vi "scope_stats.vi"(0 "Data Save":path[](array[path]), 1 "Seq":string, 4 "Save Array":bool[](array[boolean]), 5 "ext":string=".ch_a#", 6 "Repeat":u32=5, 7 "Save All":bool, 8 "Waveform Data":waveform(dbl)[](graph)=[{"t0"=timestamp(1.749999999999907e-07 s since 1904-01-01), "dt"=1e-10, "Y"=array[1000 elements]}]) -> (3 "Stats":T1(array[cluster]))   [LabVIEW 2013]
uses:
  Acquisition/statistics.ctl
  <vilib>/Utility/file.llb/Write To Spreadsheet File (string).vi
  <vilib>/Analysis/NI_AALBase.lvlib
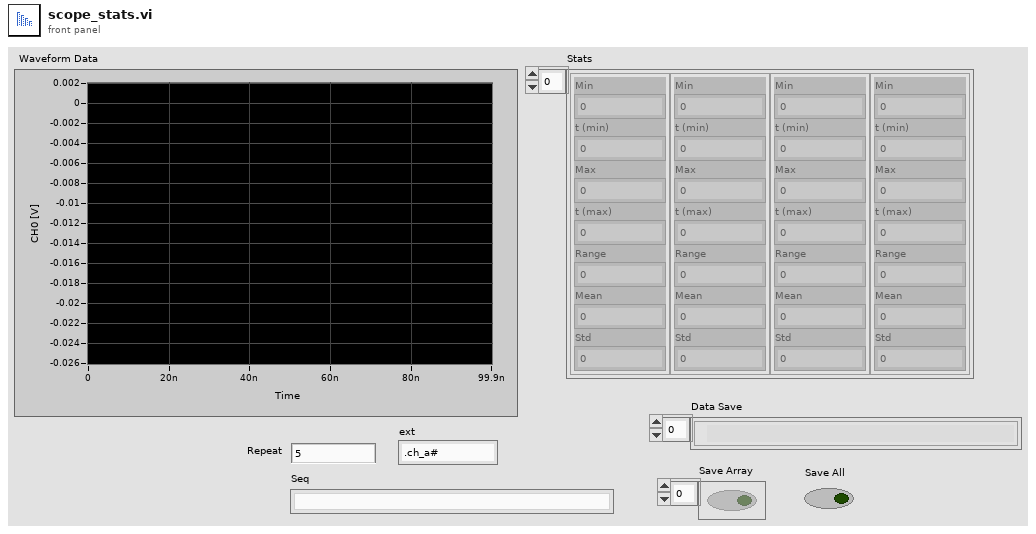
[diagram p1: front panel]
types:
  T1 = cluster{"Min":dbl, "t (min)":dbl, "Max":dbl, "t (max)":dbl, "Range":dbl, "Mean":dbl, "Std":dbl}[]
  T2 = typedef "statistics.ctl" = cluster{"min":dbl, "t_min":dbl, "max":dbl, "t_max":dbl, "range":dbl, "mean":dbl, "stdev":dbl}
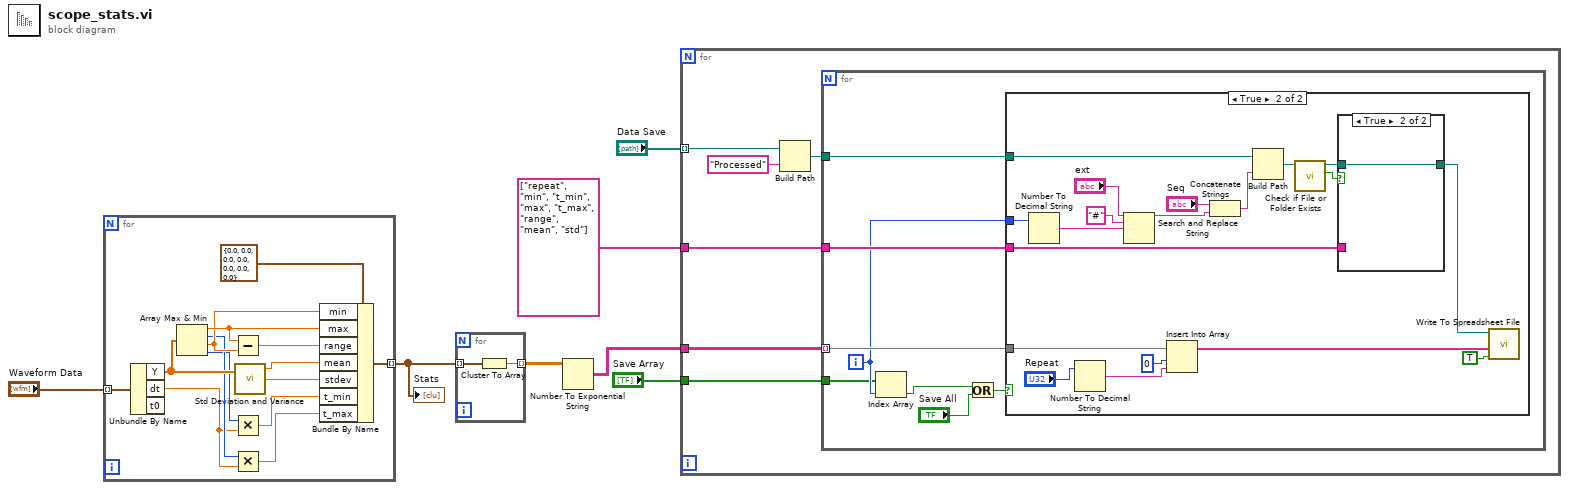
[diagram p0: block diagram]
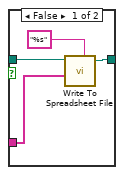
[diagram p3: hidden frame]
diagram:
  n1 = for {
    tunnel: "Waveform Data" -> [w21] mode=indexing
    tunnel: [w14] -> w6 mode=indexing
    n2 = Unbundle By Name(w21) -> ("Y"=w15:dbl[], "dt"=w10:dbl)  [unwired: 1 out]
    n3 = Array Max & Min(array=w15) -> (max value=w20:dbl, max index (indices)=w13:i32, min value=w19:dbl, min index (indices)=w11:i32)
    n4 = Subtract(x=w20, y=w19) -> (x-y=w18:dbl)
    n5 = Multiply(x=w11, y=w10) -> (x*y=w9:dbl)
    n6 = Multiply(x=w13, y=w10) -> (x*y=w12:dbl)
    n7 = call <vilib>:"Std Deviation and Variance.vi"("X"=w15) -> ("mean"=w17:dbl, "standard deviation"=w16:dbl)  [unwired: 1 in, 1 out]
    n8 = Bundle By Name(cluster=T2 {"min"=0.0, "t_min"=0.0, "max"=0.0, "t_max"=0.0, "range"=0.0, "mean"=0.0, "stdev"=0.0} ("info"), "min"=w19, "max"=w20, "range"=w18, "mean"=w17, "stdev"=w16, "t_min"=w9, "t_max"=w12) -> (w14:T2)
  }
  "Stats" <- w6
  n9 = for {
    tunnel: w6 -> [w23] mode=indexing
    tunnel: [w22] -> w4 mode=indexing
    n10 = Cluster To Array(cluster=w23) -> (array=w22:dbl[])
  }
  n11 = Number To Exponential String(number=w4) -> (E-format string=w3:string[][])  [unwired: 3 in]
  n12 = for {
    tunnel: "Data Save" -> [w27] mode=indexing
    tunnel: w3 -> [w26]
    tunnel: string[] ["repeat", "min", "t_min", "max", "t_max", "range", "mean", "std"] ("Headers") -> [w25]
    tunnel: "Save Array" -> [w24]
    n13 = Build Path(base path=w27, name or relative path="Processed") -> (appended path=w28:path)
    n14 = for {
      tunnel: w28 -> [w37]
      tunnel: w26 -> [w36] mode=indexing
      tunnel: w25 -> [w35]
      tunnel: w24 -> [w31]
      i -> [w32]
      n15 = Index Array(array=w31, index=w32) -> (element=w30:bool)
      n16 = Or(x=w30, y="Save All") -> (x .or. y?=w33:bool)
      n17 = case shown="True" w33 {
        tunnel: w37 -> [_ w56]
        tunnel: w32 -> [_ w54]
        tunnel: w36 -> [_ w47]
        tunnel: w35 -> [_ w45]
        frame False {
        }
        frame True {
          n18 = Number To Decimal String(number=w54) -> (decimal integer string=w53:string)  [unwired: 1 in]
          n19 = Number To Decimal String(number="Repeat") -> (decimal integer string=w48:string)  [unwired: 1 in]
          n20 = Search and Replace String(input string="ext", search string="#", replace string=w53) -> (result string=w40:string)  [unwired: 5 in, 3 out]
          n21 = Insert Into Array(array=w47, index=0, new element=w48) -> (w42:string[])
          n22 = Concatenate Strings("Seq", w40) -> (w38:string)
          n23 = Build Path(base path=w56, name or relative path=w38) -> (appended path=w51:path)
          n24 = call <vilib>:"Check if File or Folder Exists.vi"("path"=w51) -> ("file or folder exists?"=w50:bool, "dup path"=w44:path)  [unwired: 8 in, 1 out]
          n25 = case shown="True" w50 {
            tunnel: w45 -> [w60 _]
            tunnel: w44 -> [w58 w61]
            tunnel: [w57 w61] -> w43
            frame False {
              n26 = call-poly <vilib>:"Write To Spreadsheet File.vi"("format (%s)"="%s", "1D data"=w60, "file path (dialog if empty)"=w58) -> ("new file path (Not A Path if cancelled)"=w57:path)  [unwired: 5 in]
            }
            frame True {
            }
          }
          n27 = call-poly <vilib>:"Write To Spreadsheet File.vi"("append to file? (new file:F)"=TRUE, "1D data"=w42, "file path (dialog if empty)"=w43) -> ()  [unwired: 5 in, 1 out]
        }
      }
    }
  }
